vi "mul_18x18_dc_ht_rnd.vi"(10 "Signal":fxp<+/-,18,16>=32.0, 11 "coeff":fxp<+/-,18,2>=0.5) -> (1 "out":fxp<+/-,24,16>)   [LabVIEW 2018]
uses:
  <vilib>/rvi/FXPMathLib/basic elements/DSP48E/simVIs/niFpgaDsp48eSimulationState.ctl
  <vilib>/rvi/FXPMathLib/basic elements/DSP48E/subVIs/niFpgaDsp48eType.ctl
  <vilib>/rvi/FXPMathLib/basic elements/DSP48E/subVIs/niFpgaDsp48eAlumodeOpmodeCarryinselState.ctl
  <vilib>/rvi/FXPMathLib/basic elements/DSP48E/subVIs/niFpgaDsp48eUseMultiplierState.ctl
  <vilib>/rvi/FXPMathLib/basic elements/DSP48E/subVIs/niFpgaDsp48eLogicUnitModeState.ctl
  <vilib>/rvi/FXPMathLib/basic elements/DSP48E/subVIs/niFpgaDsp48eSelectPatternState.ctl
  <vilib>/rvi/FXPMathLib/basic elements/DSP48E/subVIs/niFpgaDsp48eSelectMaskState.ctl
  <vilib>/rvi/FXPMathLib/basic elements/DSP48E/subVIs/niFpgaDsp48eAutoresetState.ctl
  <vilib>/rvi/FXPMathLib/basic elements/DSP48E/simVIs/niFpgaDsp48eResets.ctl
  <vilib>/rvi/FXPMathLib/basic elements/DSP48E/simVIs/niFpgaDsp48eRegisters.ctl
  <vilib>/rvi/FXPMathLib/basic elements/DSP48E/simVIs/niFpgaDsp48eCheckMode.vi
  <vilib>/rvi/FXPMathLib/basic elements/DSP48E/simVIs/niFpgaDsp48eReportInvalidMode.vi
  <vilib>/rvi/FXPMathLib/basic elements/DSP48E/simVIs/niFpgaDsp48eSimBundleEnables.vi
  <vilib>/rvi/FXPMathLib/basic elements/DSP48E/simVIs/niFpgaDsp48eSimMultiplier.vi
  <vilib>/rvi/FXPMathLib/basic elements/DSP48E/simVIs/niFpgaDsp48eSimArithmetic.vi
  <vilib>/rvi/FXPMathLib/basic elements/DSP48E/simVIs/niFpgaDsp48eSimPatternDetect.vi
  <vilib>/rvi/FXPMathLib/basic elements/DSP48E/simVIs/niFpgaDsp48eSimP.vi
  <vilib>/rvi/FXPMathLib/basic elements/DSP48E/simVIs/niFpgaDsp48eSimUpdateState.vi
  <vilib>/rvi/FXPMathLib/basic elements/DSP48E/XNode/niFpgaDsp48e.xnode
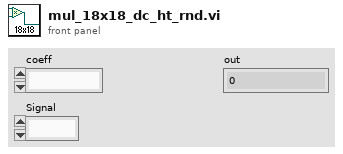
[diagram p1: front panel]
types:
  T1 = cluster{"Boolean array[0]":bool, "Boolean array[1]":bool, "Boolean array[2]":bool, "Boolean array[3]":bool, "Boolean array[4]":bool, "Boolean array[5]":bool, "Boolean array[6]":bool, "Boolean array[7]":bool, "Boolean array[8]":bool, "Boolean array[9]":bool, "Boolean array[10]":bool, "Boolean array[11]":bool, "Boolean array[12]":bool, "Boolean array[13]":bool, "Boolean array[14]":bool, "Boolean array[15]":bool, "Boolean array[16]":bool, "Boolean array[17]":bool}
  T2 = cluster{"Boolean array[0]":bool, "Boolean array[1]":bool, "Boolean array[2]":bool, "Boolean array[3]":bool, "Boolean array[4]":bool, "Boolean array[5]":bool, "Boolean array[6]":bool, "Boolean array[7]":bool, "Boolean array[8]":bool, "Boolean array[9]":bool, "Boolean array[10]":bool, "Boolean array[11]":bool, "Boolean array[12]":bool, "Boolean array[13]":bool, "Boolean array[14]":bool, "Boolean array[15]":bool, "Boolean array[16]":bool, "Boolean array[17]":bool, "Boolean array[18]":bool, "Boolean array[19]":bool, "Boolean array[20]":bool, "Boolean array[21]":bool, "Boolean array[22]":bool, "Boolean array[23]":bool, "Boolean array[24]":bool, "Boolean array[25]":bool, "Boolean array[26]":bool, "Boolean array[27]":bool, "Boolean array[28]":bool, "Boolean array[29]":bool, "Boolean array[30]":bool, "Boolean array[31]":bool, "Boolean array[32]":bool, "Boolean array[33]":bool, "Boolean array[34]":bool, "Boolean array[35]":bool, "Boolean array[36]":bool, "Boolean array[37]":bool, "Boolean array[38]":bool, "Boolean array[39]":bool, "Boolean array[40]":bool, "Boolean array[41]":bool, "Boolean array[42]":bool, "Boolean array[43]":bool, "Boolean array[44]":bool, "Boolean array[45]":bool, "Boolean array[46]":bool, "Boolean array[47]":bool}
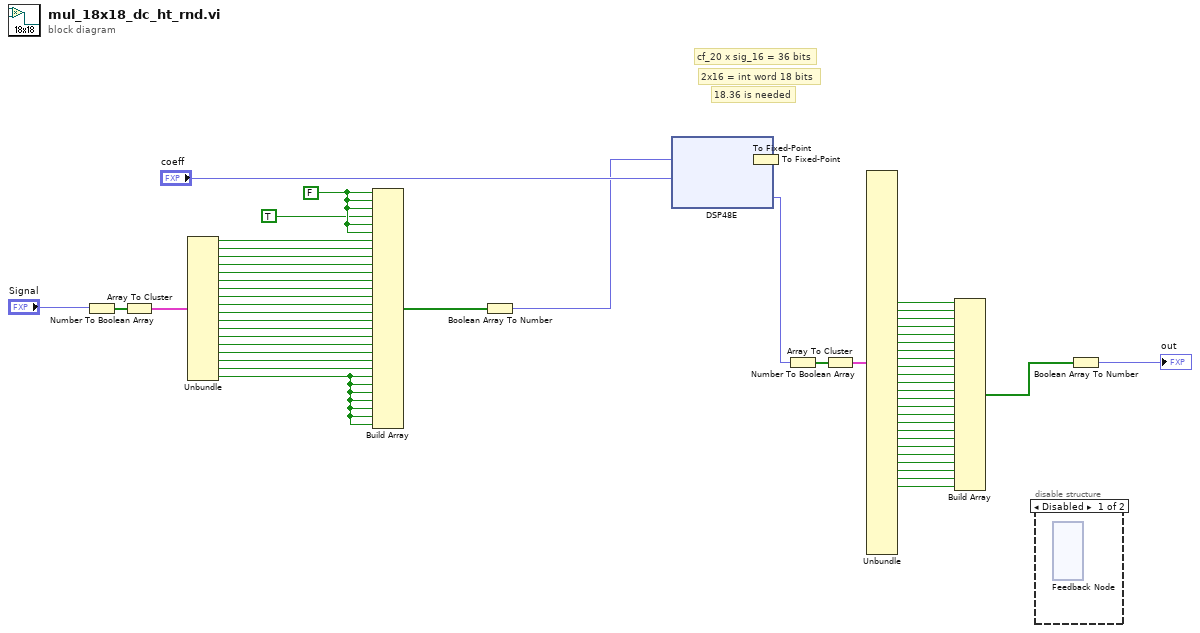
[diagram p0: block diagram]
diagram:
  w4 = FALSE ("Boolean array[0]")
  # "18.36 is needed"
  # "2x16 = int word 18 bits"
  # "cf_20 x sig_16 = 36 bits"
  n1 = Number To Boolean Array(number="Signal") -> (Boolean array=w36:bool[])
  n2 = Array To Cluster(array=w36) -> (cluster=w23:T1)
  n3 = Unbundle(w23) -> ("Boolean array[0]"=w5:bool, "Boolean array[1]"=w6:bool, "Boolean array[2]"=w7:bool, "Boolean array[3]"=w8:bool, "Boolean array[4]"=w9:bool, "Boolean array[5]"=w10:bool, "Boolean array[6]"=w11:bool, "Boolean array[7]"=w12:bool, "Boolean array[8]"=w13:bool, "Boolean array[9]"=w14:bool, "Boolean array[10]"=w15:bool, "Boolean array[11]"=w16:bool, "Boolean array[12]"=w17:bool, "Boolean array[13]"=w18:bool, "Boolean array[14]"=w19:bool, "Boolean array[15]"=w20:bool, "Boolean array[16]"=w21:bool, "Boolean array[17]"=w22:bool)
  n4 = Build Array(w4, w4, w4, TRUE ("Boolean array[0]"), w4, w4, w5, w6, w7, w8, w9, w10, w11, w12, w13, w14, w15, w16, w17, w18, w19, w20, w21, w22, w22, w22, w22, w22, w22, w22) -> (w40:bool[])
  n5 = Boolean Array To Number(Boolean array=w40) -> (number=w34:fxp<+/-,30,22>)
  n6 = To Fixed-Point(number=w34) -> (fixed-point=w1:fxp<+/-,30,22>)  [unwired: 1 in]
  n7 = To Fixed-Point(number=w1) -> (fixed-point=w2:fxp<+/-,25,17>)  [unwired: 1 in]
  n8 = xnode ("DSP48E")("a"=w2, "b"="coeff") -> ("p"=w46:fxp<+/-,48,16>)
  n9 = Number To Boolean Array(number=w46) -> (Boolean array=w37:bool[])
  n10 = Array To Cluster(array=w37) -> (cluster=w57:T2)
  n11 = Unbundle(w57) -> ("Boolean array[16]"=w27:bool, "Boolean array[17]"=w26:bool, "Boolean array[18]"=w33:bool, "Boolean array[19]"=w32:bool, "Boolean array[20]"=w31:bool, "Boolean array[21]"=w30:bool, "Boolean array[22]"=w29:bool, "Boolean array[23]"=w28:bool, "Boolean array[24]"=w50:bool, "Boolean array[25]"=w51:bool, "Boolean array[26]"=w52:bool, "Boolean array[27]"=w53:bool, "Boolean array[28]"=w54:bool, "Boolean array[29]"=w55:bool, "Boolean array[30]"=w56:bool, "Boolean array[31]"=w47:bool, "Boolean array[32]"=w48:bool, "Boolean array[33]"=w49:bool, "Boolean array[34]"=w45:bool, "Boolean array[35]"=w44:bool, "Boolean array[36]"=w39:bool, "Boolean array[37]"=w38:bool, "Boolean array[38]"=w24:bool, "Boolean array[39]"=w25:bool)  [unwired: 24 out]
  n12 = Build Array(w27, w26, w33, w32, w31, w30, w29, w28, w50, w51, w52, w53, w54, w55, w56, w47, w48, w49, w45, w44, w39, w38, w24, w25) -> (w43:bool[])
  n13 = disable-structure shown="Disabled" {
    frame Disabled {
      n14 = feedback #1() -> ()  [unwired: 2 in]
      n15 = feedback-in #1() -> ()  [unwired: 1 in, 1 out]
    }
    frame Enabled {
    }
  }
  n16 = Boolean Array To Number(Boolean array=w43) -> (number=→"out":fxp<+/-,24,16>)
